vi "Remote Auto VideoMode.vi"(2 "Resolution":T1=1 items=["Low", "Med", "High", "Max."], 3 "Camera":T2="Travcam") -> (0 "Error out":errorcluster, 1 "VideoMode":u32)   [LabVIEW 2015]
uses:
  Camera enum/Camera enum.ctl
  Camera enum/Camera resolution.ctl
  Globals/CamServer global.vi
panel:
  # "PN 27/08/2015"
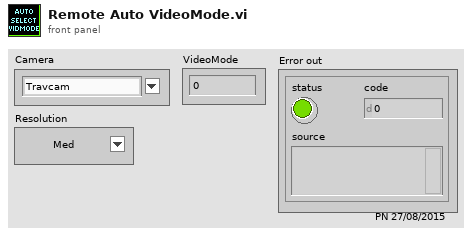
[diagram p1: front panel]
types:
  T1 = typedef "Camera resolution.ctl" = u8
  T2 = typedef "Camera enum.ctl" = string
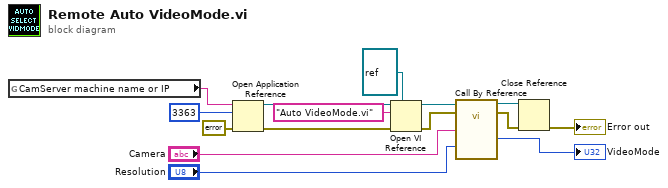
[diagram p0: block diagram]
diagram:
  n1 = global read "CamServer global.vi" "CamServer machine name or IP"() -> (w9:string)
  n2 = Open Application Reference(8:errorcluster {"status"=FALSE, "code"=0, "source"=""} ("error in (no error)"), 10:u16 3363 ("port"), 11:w9) -> (0:w5:errorcluster, 3:w6:refnum<vi>)  [unwired: 1 in]
  n3 = Open VI Reference(type specifier VI Refnum (for type only)=refnum<vi> refnum, application reference (local)=w6, vi path="Auto VideoMode.vi" ("machine name"), error in (no error)=w5) -> (vi reference=w13:refnum<vi>, error out=w12:errorcluster)  [unwired: 2 in]
  n4 = call-by-ref "?"(reference=w13, error in=w12, "Resolution"="Resolution", "Camera"="Camera") -> (reference out=w11:refnum<vi>, error out=w10:errorcluster, "VideoMode"=→"VideoMode":u32)
  n5 = Close Reference(reference=w11, error in (no error)=w10) -> (error out=→"Error out":errorcluster)
